vi "CoordGen.vi"() -> (3 "Coord":dbl[][](array[numeric]))   [LabVIEW 2020]
panel:
  out "size(s)":i32[](array[numeric])
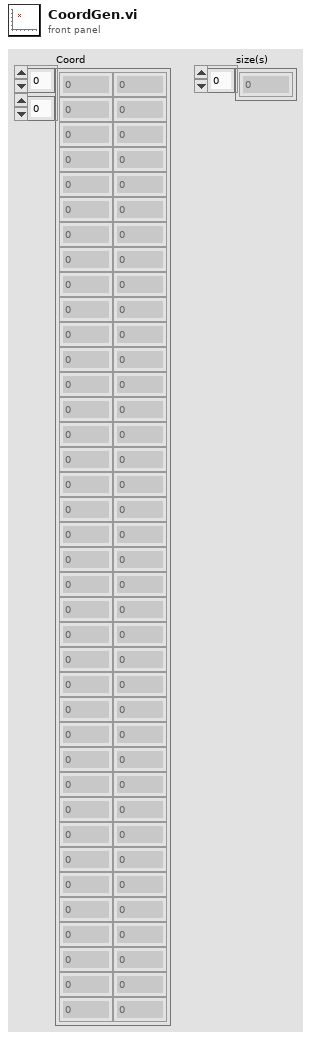
[diagram p1: front panel]
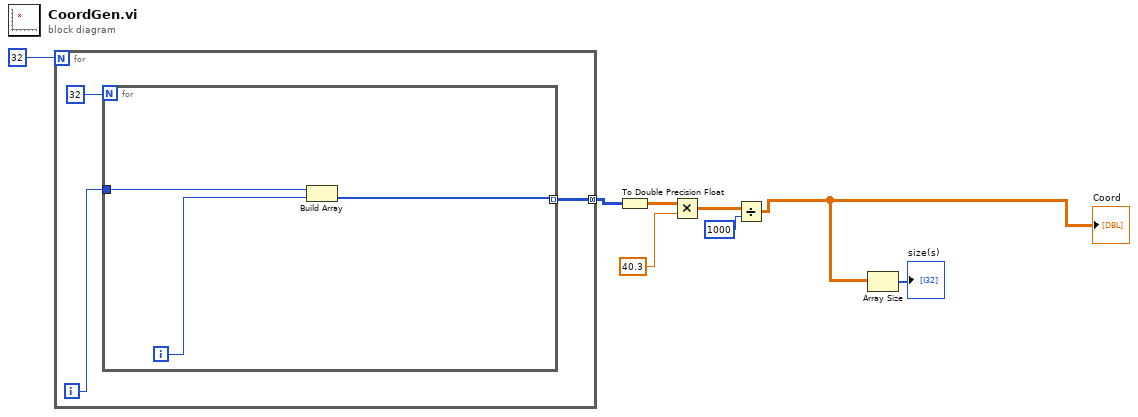
[diagram p0: block diagram]
diagram:
  n1 = for {
    N: 32 -> [_]
    tunnel: [w10] -> w4 mode=concatenating
    i -> [w11]
    n2 = for {
      N: 32 -> [_]
      tunnel: w11 -> [w13]
      tunnel: [w12] -> w10 mode=indexing
      i -> [w14]
      n3 = Build Array(w13, w14) -> (w12:i32[])
    }
  }
  n4 = To Double Precision Float(number=w4) -> (double precision float=w3:dbl[][])
  n5 = Multiply(x=w3, y=40.3) -> (x*y=w6:dbl[][])
  n6 = Divide(x=w6, y=1000) -> (x/y=w2:dbl[][])
  "Coord" <- w2
  n7 = Array Size(array=w2) -> (size(s)=→"size(s)":i32[])
